vi "pickRobotsVSS.vi"(8 "error in (no error)":errorcluster, 11 "Game in":refnum<class "Game.lvclass">) -> (0 "error out":errorcluster, 3 "Game out":refnum<class "Game.lvclass">)   [LabVIEW 2020, in "Game.lvclass"]
uses:
  Game.lvclass
  Game.lvclass/Game.ctl
  Referee_class/Referee.lvclass/Referee.ctl
  Team_class/Team.lvclass/Team.ctl
  Robot_class/roles.ctl
  Robot_class/Robot.lvclass/Robot.ctl
  Role_class/Role.lvclass/Role.ctl
  HaltPlay_class/HaltPlay.lvclass/HaltPlay.ctl
  TimeoutPlay_class/TimeoutPlay.lvclass/TimeoutPlay.ctl
  Robot_class/Write role.vi
  Role_class/Write RobotRef.vi
  HaltPlay_class/Read Roles.vi
  HaltPlay_class/Write Roles.vi
  TimeoutPlay_class/Read Roles.vi
  TimeoutPlay_class/Write Roles.vi
  Read KeeperTeam.vi
  Read AllyRef.vi
  Read Referee.vi
  Read TestMode IDs.vi
  Referee_class/Read our_goalie_id.vi
  Team_class/Read RobotRef.vi
  Team_class/Write RobotRef.vi
  Write KeeperTeam.vi
  Ally_class/Ally.lvclass
  C:/Users/lucio/Desktop/Horie/ROBOIME/VSS_AI/Team_class/Team.lvclass
  KeeperRoleVSS_class/KeeperRoleVSS.lvclass
  C:/Users/lucio/Desktop/Horie/ROBOIME/VSS_AI/Role_class/Role.lvclass
  NormalAttackerRoleVSS_class/NormalAttackerRoleVSS.lvclass
  DefenderAreaRoleVSS_class/DefenderAreaRoleVSS.lvclass
  HaltRole_class/HaltRole.lvclass
  GoalKickKeeperRoleVSS_class/GoalKickKeeperRoleVSS.lvclass
  GoAndKickRoleVSS_class/GoAndKickRoleVSS.lvclass
  BallChallengerAttackerRoleVSS_class/BallChallengerAttackerRoleVSS.lvclass
  TimeoutRole_class/TimeoutRole.lvclass
  Referee_class/Referee.lvclass
  Playbook_class/Playbook.lvclass
  Robot_class/Robot.lvclass
  PreparePenaltyAllyPlayVSS_class/PreparePenaltyAllyPlayVSS.lvclass
  HaltPlay_class/HaltPlay.lvclass
  DeadBallPlayVSS_class/DeadBallPlayVSS.lvclass
  NormalGamePlayVSS_class/NormalGamePlayVSS.lvclass
  BallChallengePlayVSS_class/BallChallengePlayVSS.lvclass
  PenaltyEnemyPlayVSS_class/PenaltyEnemyPlayVSS.lvclass
  TimeoutPlay_class/TimeoutPlay.lvclass
  KickPenaltyAllyPlayVSS_class/KickPenaltyAllyPlayVSS.lvclass
  PreparePenaltyEnemyPlayVSS_class/PreparePenaltyEnemyPlayVSS.lvclass
  PrepareKickoffAllyPlayVSS_class/PrepareKickoffAllyPlayVSS.lvclass
  PrepareKickoffEnemyPlayVSS_class/PrepareKickoffEnemyPlayVSS.lvclass
  PrepareGoalKickAllyPlayVSS_class/PrepareGoalKickAllyPlayVSS.lvclass
  PrepareGoalKickEnemyPlayVSS_class/PrepareGoalKickEnemyPlayVSS.lvclass
  PrepareFreeBallPlayVSS_class/PrepareFreeBallPlayVSS.lvclass
  FreeBallPlayVSS_class/FreeBallPlayVSS.lvclass
  GoalKickAllyPlayVSS_class/GoalKickAllyPlayVSS.lvclass
  GoalKickEnemyPlayVSS_class/GoalKickEnemyPlayVSS.lvclass
  KickoffAllyPlayVSS_class/KickoffAllyPlayVSS.lvclass
  KickoffEnemyPlayVSS_class/KickoffEnemyPlayVSS.lvclass
  StopPlayVSS_class/StopPlayVSS.lvclass
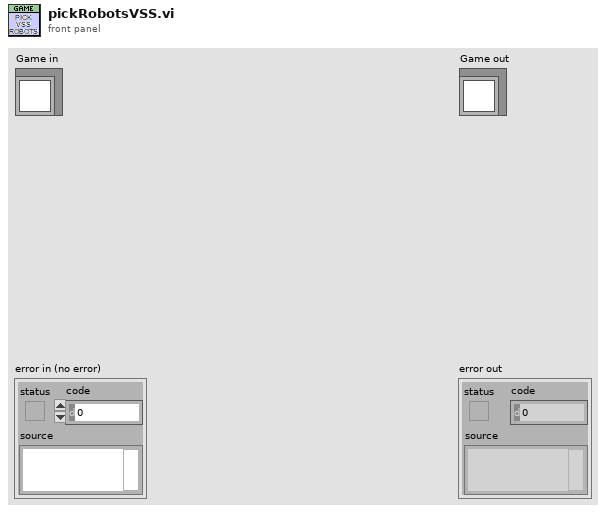
[diagram p1: front panel]
types:
  T1 = typedef "roles.ctl" = enum16{"BallChallengerAttackerVSS", "NormalAttackerVSS", "AttackerAimGoalVSS", "DefenderAreaVSS", "KeeperVSS", "Tabler", "TableFinalizer", "PrepareRollToPassRoller", "PrepareRollToPassReceiver", "SimplePassRoll", "SimplePassRollReceiver", "PenaltyDefense", "PreparePassReceiver 2", "PreparePassReceiver 1", "PassObserver", "Timeout", "Goto", "ZigZag", "None", "BallOutOfField", "DefenderArea", "Duelist", "AttackerStop", "FollowAttacker", "KeeperRole", "KickPenalty", "AttackerAimGoal", "AttackerBlock", "Marker", "Halt", "Shoot", "PassKicker", "PassReceiver", "TestRole", "PenaltyAttacker"}
  T2 = enum16{"FreeBall", "PrepareFreeBall", "GoalKickEnemy", "GoalKickAlly", "KickoffAlly", "KickoffEnemy", "PrepareGoalKickEnemy", "PrepareGoalKickAlly", "Stop", "PrepareKickoffEnemy", "PrepareKickoffAlly", "PreparePenaltyEnemy", "Timeout", "DeadBall", "NormalGame", "KickPenaltyAlly", "PenaltyEnemy", "BallChallenge", "PreparePenaltyAlly", "Halt"}
  T3 = cluster{"PreparePenaltyAllyPlayVSS":refnum<class "PreparePenaltyAllyPlayVSS.lvclass">, "HaltPlay":refnum<class "HaltPlay.lvclass">, "DeadBallPlayVSS":refnum<class "DeadBallPlayVSS.lvclass">, "NormalGamePlayVSS":refnum<class "NormalGamePlayVSS.lvclass">, "BallChallengePlayVSS":refnum<class "BallChallengePlayVSS.lvclass">, "PenaltyEnemyPlayVSS":refnum<class "PenaltyEnemyPlayVSS.lvclass">, "TimeoutPlay":refnum<class "TimeoutPlay.lvclass">, "KickPenaltyAllyPlayVSS":refnum<class "KickPenaltyAllyPlayVSS.lvclass">, "PreparePenaltyEnemyPlayVSS":refnum<class "PreparePenaltyEnemyPlayVSS.lvclass">, "PrepareKickoffAllyPlayVSS":refnum<class "PrepareKickoffAllyPlayVSS.lvclass">, "PrepareKickoffEnemyPlayVSS":refnum<class "PrepareKickoffEnemyPlayVSS.lvclass">, "PrepareGoalKickAllyPlayVSS":refnum<class "PrepareGoalKickAllyPlayVSS.lvclass">, "PrepareGoalKickEnemyPlayVSS":refnum<class "PrepareGoalKickEnemyPlayVSS.lvclass">, "PrepareFreeBallPlayVSS":refnum<class "PrepareFreeBallPlayVSS.lvclass">, "FreeBallPlayVSS":refnum<class "FreeBallPlayVSS.lvclass">, "GoalKickAllyPlayVSS":refnum<class "GoalKickAllyPlayVSS.lvclass">, "GoalKickEnemyPlayVSS":refnum<class "GoalKickEnemyPlayVSS.lvclass">, "KickoffAllyPlayVSS":refnum<class "KickoffAllyPlayVSS.lvclass">, "KickoffEnemyPlayVSS":refnum<class "KickoffEnemyPlayVSS.lvclass">, "StopPlayVSS":refnum<class "StopPlayVSS.lvclass">}
  T4 = cluster{"NormalAttackerRoleVSS":refnum<class "NormalAttackerRoleVSS.lvclass">, "KeeperRoleVSS":refnum<class "KeeperRoleVSS.lvclass">, "DefenderAreaRoleVSS":refnum<class "DefenderAreaRoleVSS.lvclass">}
  T5 = cluster{"HaltRole K":refnum<class "HaltRole.lvclass">, "HaltRole D":refnum<class "HaltRole.lvclass">, "HaltRole A":refnum<class "HaltRole.lvclass">}
  T6 = cluster{"KeeperRoleVSS":refnum<class "KeeperRoleVSS.lvclass">, "DefenderAreaRoleVSS":refnum<class "DefenderAreaRoleVSS.lvclass">, "HaltRole":refnum<class "HaltRole.lvclass">}
  T7 = cluster{"HaltRole A":refnum<class "HaltRole.lvclass">, "HaltRole D":refnum<class "HaltRole.lvclass">, "GoalKickKeeperRoleVSS":refnum<class "GoalKickKeeperRoleVSS.lvclass">}
  T8 = cluster{"KeeperRoleVSS":refnum<class "KeeperRoleVSS.lvclass">, "HaltRole":refnum<class "HaltRole.lvclass">, "GoAndKickRoleVSS":refnum<class "GoAndKickRoleVSS.lvclass">}
  T9 = cluster{"KeeperRoleVSS":refnum<class "KeeperRoleVSS.lvclass">, "HaltRole A":refnum<class "HaltRole.lvclass">, "HaltRole D":refnum<class "HaltRole.lvclass">}
  T10 = cluster{"HaltRole 1":refnum<class "HaltRole.lvclass">, "HaltRole 2":refnum<class "HaltRole.lvclass">, "HaltRole 3":refnum<class "HaltRole.lvclass">, "HaltRole 4":refnum<class "HaltRole.lvclass">, "HaltRole 5":refnum<class "HaltRole.lvclass">, "HaltRole 6":refnum<class "HaltRole.lvclass">}
  T11 = cluster{"NormalAttackerRoleVSS":refnum<class "NormalAttackerRoleVSS.lvclass">, "HaltRole K":refnum<class "HaltRole.lvclass">, "HaltRole D":refnum<class "HaltRole.lvclass">}
  T12 = cluster{"HaltRole 1":refnum<class "HaltRole.lvclass">, "HaltRole 2":refnum<class "HaltRole.lvclass">, "BallChallengerAttackerRoleVSS":refnum<class "BallChallengerAttackerRoleVSS.lvclass">}
  T13 = cluster{"TimeoutRole 1":refnum<class "TimeoutRole.lvclass">, "TimeoutRole 2":refnum<class "TimeoutRole.lvclass">, "TimeoutRole 3":refnum<class "TimeoutRole.lvclass">, "TimeoutRole 4":refnum<class "TimeoutRole.lvclass">, "TimeoutRole 5":refnum<class "TimeoutRole.lvclass">, "TimeoutRole 6":refnum<class "TimeoutRole.lvclass">}
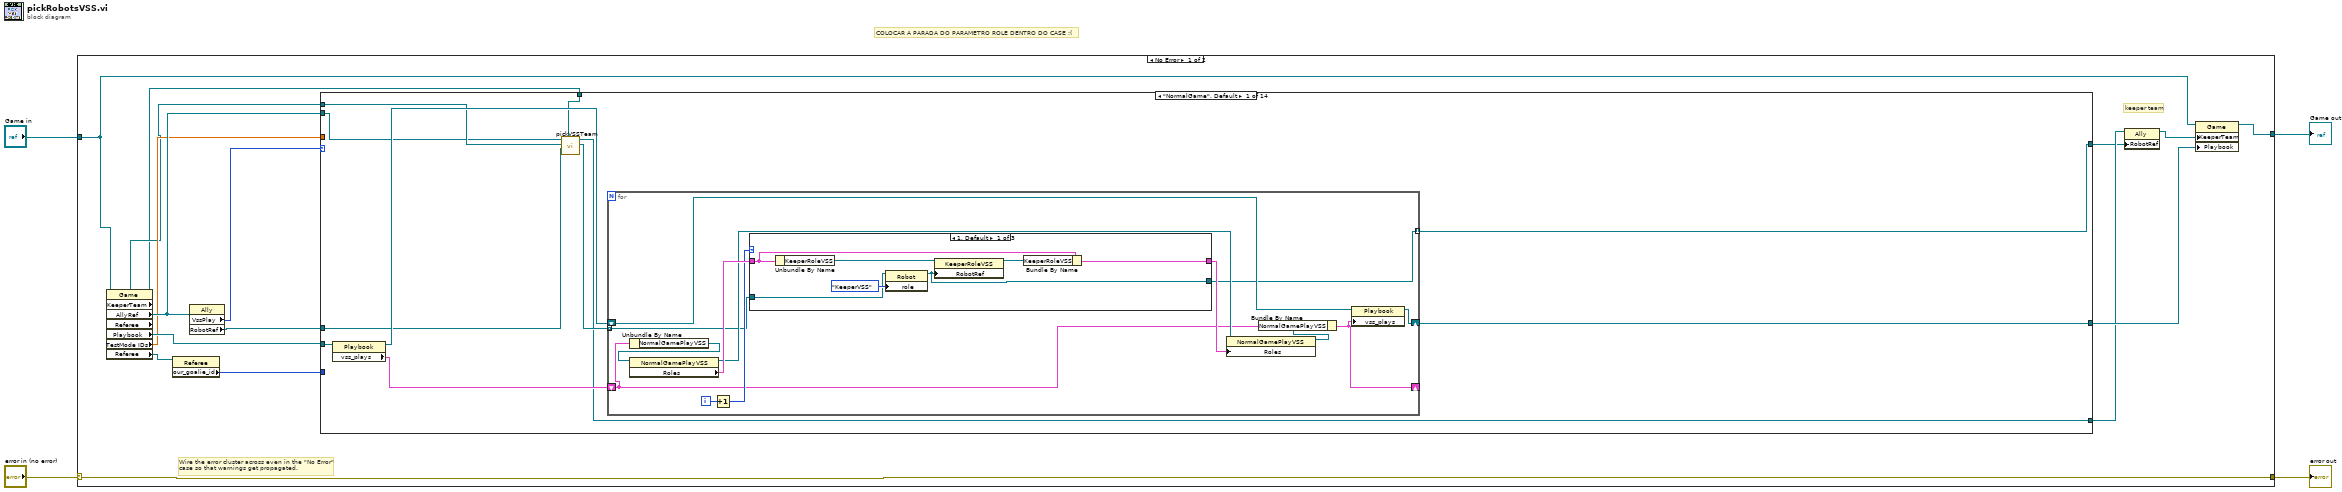
[diagram p0: block diagram]
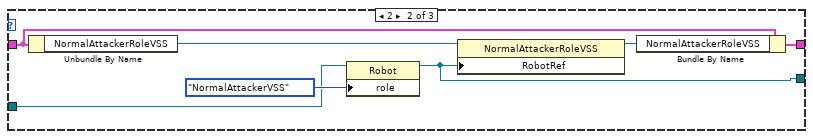
[diagram p2: hidden frame]
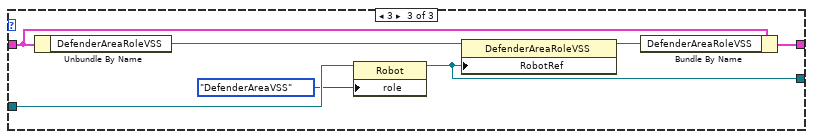
[diagram p3: hidden frame]
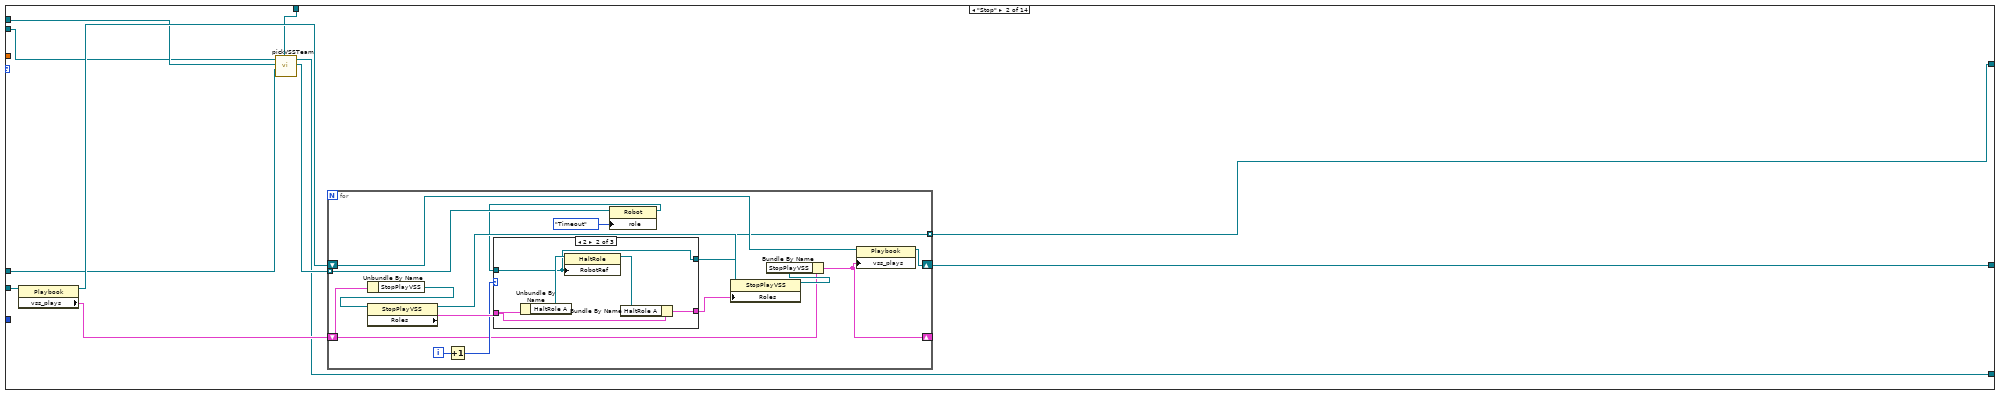
[diagram p4: hidden frame]
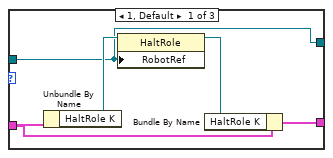
[diagram p5: hidden frame]
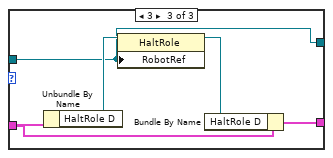
[diagram p6: hidden frame]
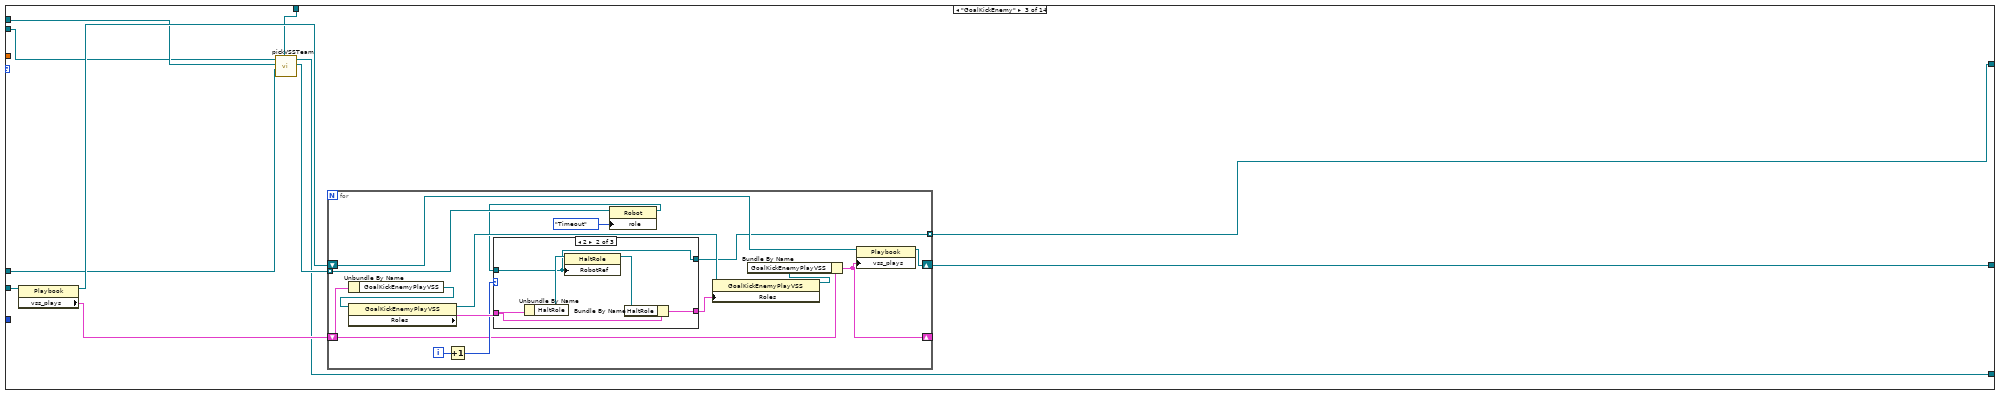
[diagram p7: hidden frame]
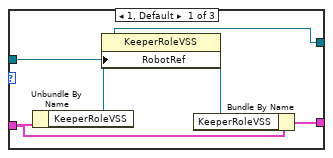
[diagram p8: hidden frame]
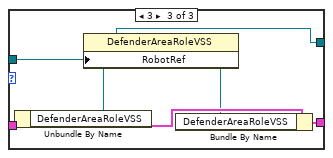
[diagram p9: hidden frame]
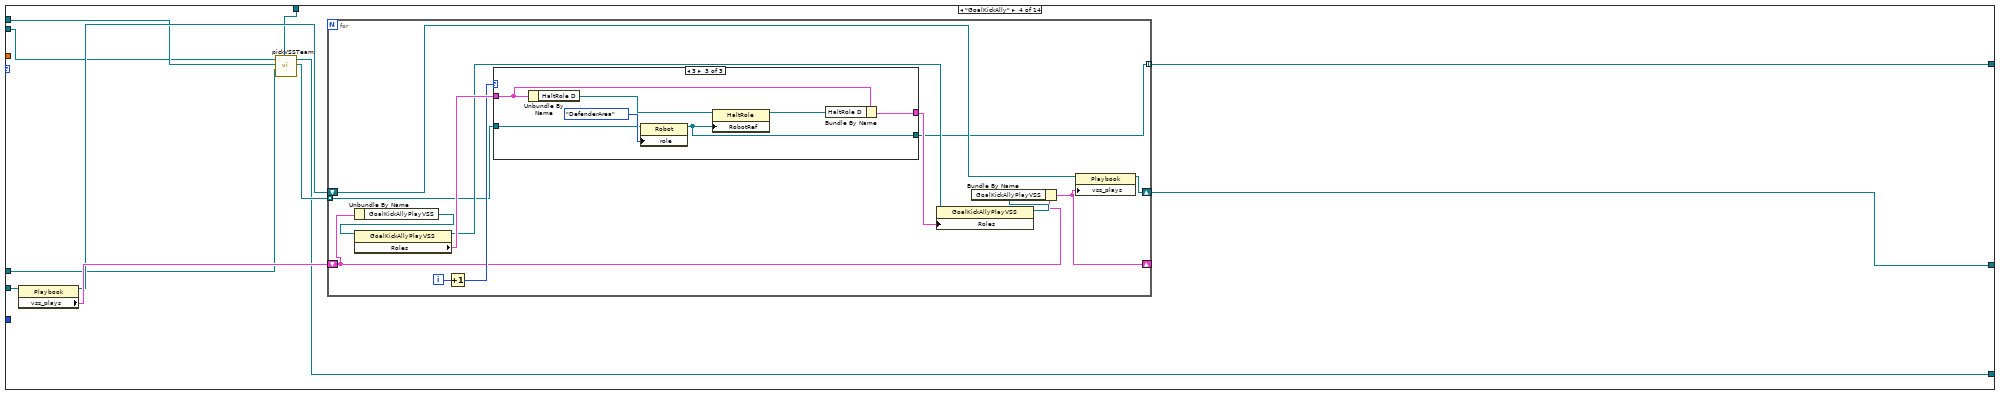
[diagram p10: hidden frame]
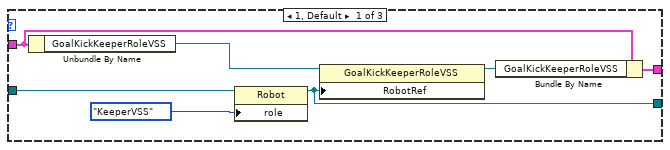
[diagram p11: hidden frame]
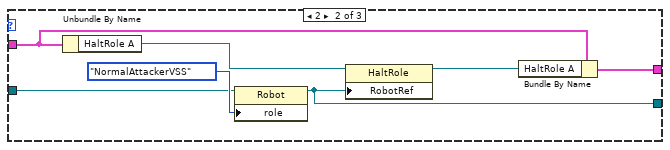
[diagram p12: hidden frame]
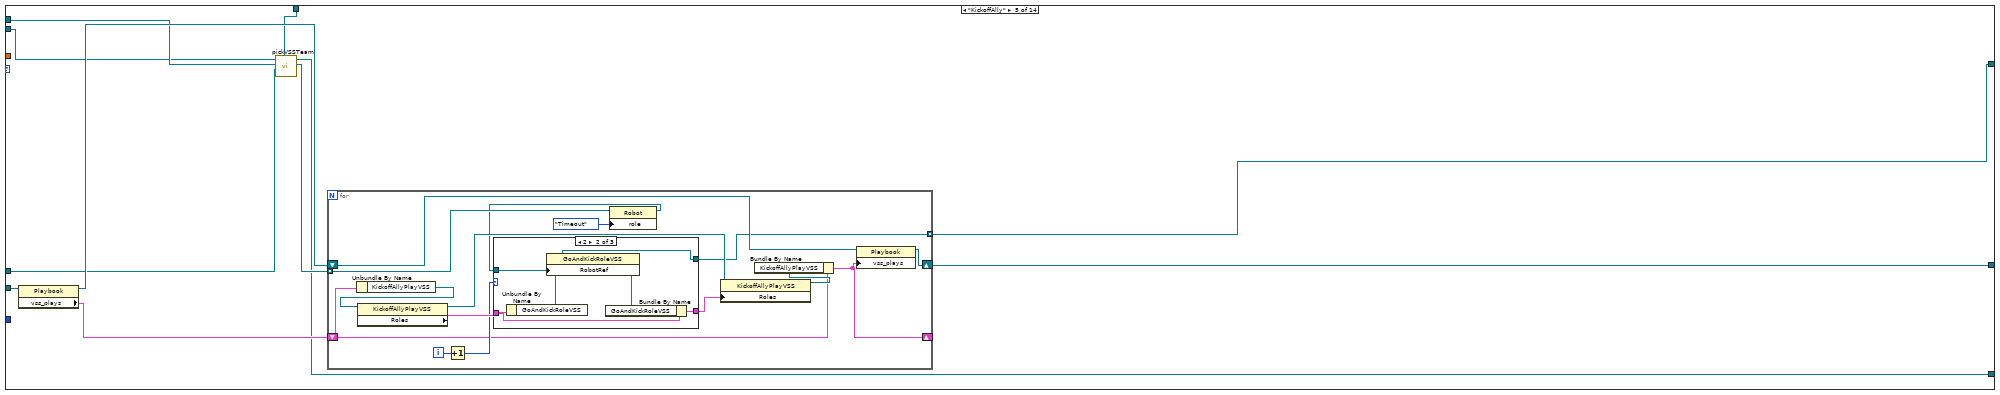
[diagram p13: hidden frame]
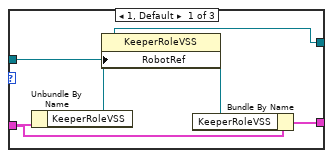
[diagram p14: hidden frame]
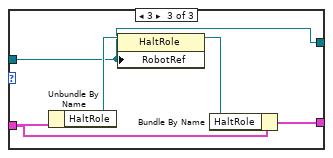
[diagram p15: hidden frame]
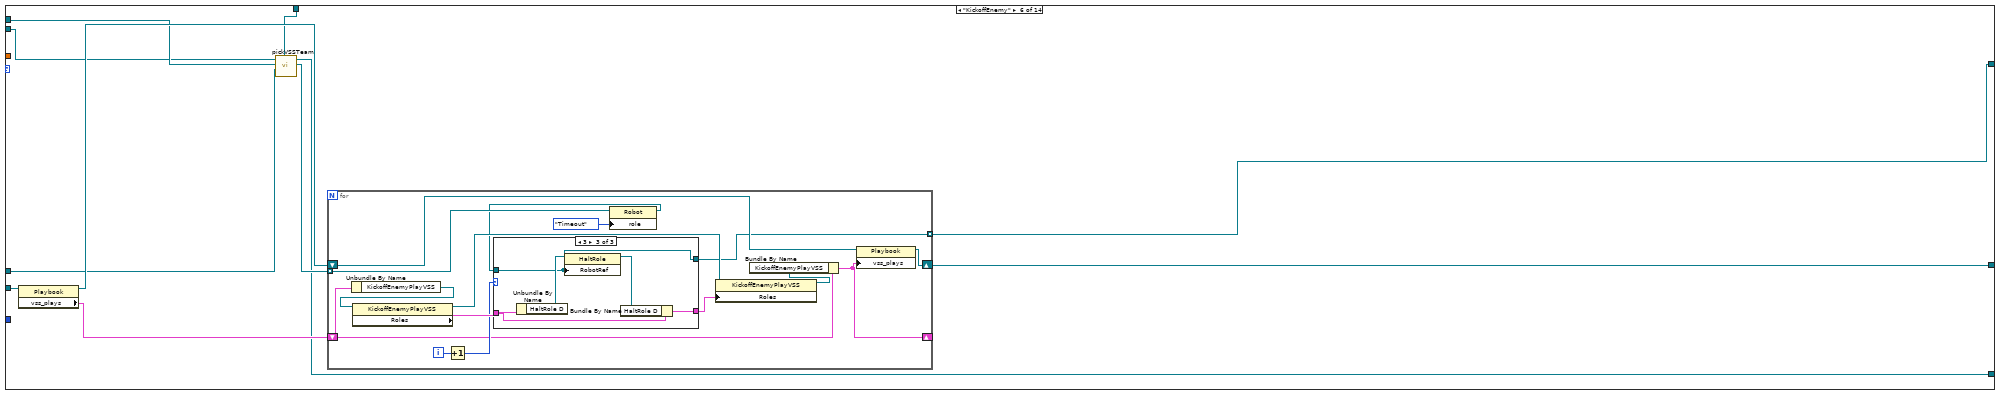
[diagram p16: hidden frame]
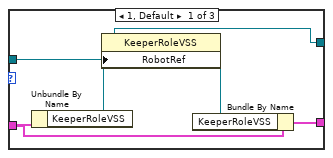
[diagram p17: hidden frame]
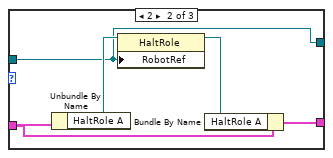
[diagram p18: hidden frame]
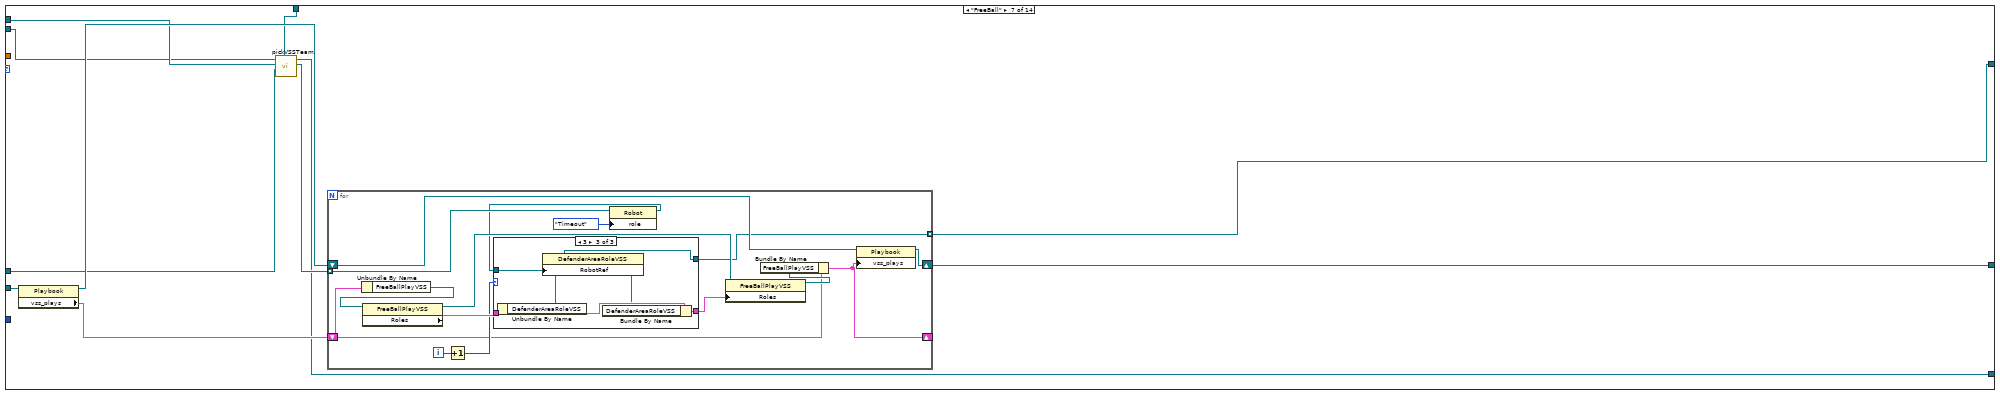
[diagram p19: hidden frame]
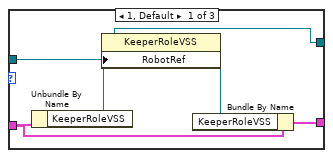
[diagram p20: hidden frame]
diagram:
  # "COLOCAR A PARADA DO PARAMETRO ROLE DENTRO DO CASE :("
  n1 = case shown="No Error" "error in (no error)" {
    selector: "error in (no error)" -> [w15 w604]
    tunnel: [w15 w604] -> w3
    tunnel: [w16 w603] -> w1
    tunnel: "Game in" -> [w18 w603]
    frame No Error {
      # "keeper team"
      # "Wire the error cluster across even in the \"No Error\"\ncase so that warnings get propagated."
      n2 = property class="Game" props=["KeeperTeam", "AllyRef", "Referee", "Playbook", "TestMode IDs", "Referee"](reference=w18) -> (reference out=w5:refnum<class "Game.lvclass">, "KeeperTeam"=w6:refnum<class "Ally.lvclass">, "AllyRef"=w12:refnum<class "Ally.lvclass">, "Playbook"=w20:refnum<class "Playbook.lvclass">, "TestMode IDs"=w9:dbl[], "Referee"=w8:refnum<class "Referee.lvclass">)  [unwired: 1 in, 2 out]
      n3 = property class="Referee"(reference=w8) -> ("our_goalie_id"=w7:i32)  [unwired: 1 in, 2 out]
      n4 = property class="Ally"(reference=w12) -> ("VssPlay"=w10:T2, "RobotRef"=w19:refnum<class "Robot.lvclass">[])  [unwired: 1 in, 2 out]
      n5 = case shown="\"NormalGame\", Default" w10 {
        tunnel: w20 -> [w31 w76 w117 w158 w203 w244 w285 w326 w367 w408 w449 w490 w531 w572]
        tunnel: w19 -> [w24 w69 w110 w151 w196 w237 w278 w319 w360 w401 w442 w483 w524 w565]
        tunnel: [w29 w74 w115 w156 w201 w242 w283 w324 w365 w406 w447 w488 w529 w570] -> w17
        tunnel: [w28 w73 w114 w155 w200 w241 w282 w323 w364 w405 w446 w487 w528 w569] -> w11
        tunnel: [w21 w66 w107 w148 w193 w234 w275 w316 w357 w398 w439 w480 w521 w562] -> w13
        tunnel: w12 -> [w25 w70 w111 w152 w197 w238 w279 w320 w361 w402 w443 w484 w525 w566]
        tunnel: w9 -> [_ _ _ _ _ _ _ _ _ _ _ _ _ _]
        tunnel: w7 -> [_ _ _ _ _ _ _ _ _ _ _ _ _ _]
        tunnel: w6 -> [w26 w71 w112 w153 w198 w239 w280 w321 w362 w403 w444 w485 w526 w567]
        tunnel: w5 -> [w23 w68 w109 w150 w195 w236 w277 w318 w359 w400 w441 w482 w523 w564]
        frame "NormalGame", Default {
          n6 = property class="Playbook"(reference=w31) -> (reference out=w27:refnum<class "Playbook.lvclass">, "vss_plays"=w30:T3)  [unwired: 1 in, 1 out]
          n7 = call "pickVSSTeam.vi"("Ally in"=w25, "OldVSSTeam"=w26, "RobotRef"=w24, "Game"=w23) -> ("Ally out"=w21:refnum<class "Ally.lvclass">, "RobotRef Out"=w22:refnum<class "Robot.lvclass">[])  [unwired: 4 in, 1 out]
          n8 = for {
            tunnel: [w34] -> w28 mode=indexing
            tunnel: w22 -> [w32] mode=indexing
            shift-right: [w39] -> w29
            shift-left: w27 -> [w40]
            shift-right: [w33] -> _
            shift-left: w30 -> [w36]
            i -> [w38]
            n9 = Unbundle By Name(w36) -> ("NormalGamePlayVSS"=w35:refnum<class "NormalGamePlayVSS.lvclass">)
            n10 = property class="NormalGamePlayVSS"(reference=w35) -> (reference out=w42:refnum<class "NormalGamePlayVSS.lvclass">, "Roles"=w44:T4)  [unwired: 1 in, 1 out]
            n11 = Increment(x=w38) -> (x+1=w37:i32)
            n12 = case shown="1, Default" w37 {
              tunnel: w44 -> [w50 w57 w64]
              tunnel: [w49 w56 w63] -> w43
              tunnel: [w45 w52 w61] -> w34
              tunnel: w32 -> [w46 w53 w60]
              frame 1, Default {
                n13 = Unbundle By Name(w50) -> ("KeeperRoleVSS"=w51:refnum<class "KeeperRoleVSS.lvclass">)
                n14 = property class="Robot"(reference=w46, "role"=roles."KeeperVSS") -> (reference out=w45:refnum<class "Robot.lvclass">)  [unwired: 1 in, 1 out]
                n15 = property class="KeeperRoleVSS"(reference=w51, "RobotRef"=w45) -> (reference out=w48:refnum<class "KeeperRoleVSS.lvclass">)  [unwired: 1 in, 1 out]
                n16 = Bundle By Name(cluster=w50, "KeeperRoleVSS"=w48) -> (w49:T4)
              }
              frame 2 {
                n17 = Unbundle By Name(w57) -> ("NormalAttackerRoleVSS"=w58:refnum<class "NormalAttackerRoleVSS.lvclass">)
                n18 = property class="Robot"(reference=w53, "role"=roles."NormalAttackerVSS") -> (reference out=w52:refnum<class "Robot.lvclass">)  [unwired: 1 in, 1 out]
                n19 = property class="NormalAttackerRoleVSS"(reference=w58, "RobotRef"=w52) -> (reference out=w55:refnum<class "NormalAttackerRoleVSS.lvclass">)  [unwired: 1 in, 1 out]
                n20 = Bundle By Name(cluster=w57, "NormalAttackerRoleVSS"=w55) -> (w56:T4)
              }
              frame 3 {
                n21 = Unbundle By Name(w64) -> ("DefenderAreaRoleVSS"=w65:refnum<class "DefenderAreaRoleVSS.lvclass">)
                n22 = property class="Robot"(reference=w60, "role"=roles."DefenderAreaVSS") -> (reference out=w61:refnum<class "Robot.lvclass">)  [unwired: 1 in, 1 out]
                n23 = property class="DefenderAreaRoleVSS"(reference=w65, "RobotRef"=w61) -> (reference out=w62:refnum<class "DefenderAreaRoleVSS.lvclass">)  [unwired: 1 in, 1 out]
                n24 = Bundle By Name(cluster=w64, "DefenderAreaRoleVSS"=w62) -> (w63:T4)
              }
            }
            n25 = property class="NormalGamePlayVSS"(reference=w42, "Roles"=w43) -> (reference out=w41:refnum<class "NormalGamePlayVSS.lvclass">)  [unwired: 1 in, 1 out]
            n26 = Bundle By Name(cluster=w36, "NormalGamePlayVSS"=w41) -> (w33:T3)
            n27 = property class="Playbook"(reference=w40, "vss_plays"=w33) -> (reference out=w39:refnum<class "Playbook.lvclass">)  [unwired: 1 in, 1 out]
          }
        }
        frame "Stop" {
          n28 = property class="Playbook"(reference=w76) -> (reference out=w72:refnum<class "Playbook.lvclass">, "vss_plays"=w75:T3)  [unwired: 1 in, 1 out]
          n29 = call "pickVSSTeam.vi"("Ally in"=w70, "OldVSSTeam"=w71, "RobotRef"=w69, "Game"=w68) -> ("Ally out"=w66:refnum<class "Ally.lvclass">, "RobotRef Out"=w67:refnum<class "Robot.lvclass">[])  [unwired: 4 in, 1 out]
          n30 = for {
            tunnel: [w79] -> w73 mode=indexing
            tunnel: w67 -> [w84] mode=indexing
            shift-right: [w86] -> w74
            shift-left: w72 -> [w87]
            shift-right: [w77] -> _
            shift-left: w75 -> [w81]
            i -> [w83]
            n31 = Unbundle By Name(w81) -> ("StopPlayVSS"=w80:refnum<class "StopPlayVSS.lvclass">)
            n32 = property class="StopPlayVSS"(reference=w80) -> (reference out=w89:refnum<class "StopPlayVSS.lvclass">, "Roles"=w91:T5)  [unwired: 1 in, 1 out]
            n33 = Increment(x=w83) -> (x+1=w82:i32)
            n34 = property class="Robot"(reference=w84, "role"=roles."Timeout") -> (reference out=w78:refnum<class "Robot.lvclass">)  [unwired: 1 in, 1 out]
            n35 = case shown="2" w82 {
              tunnel: w91 -> [w95 w100 w105]
              tunnel: [w94 w99 w104] -> w90
              tunnel: w78 -> [w92 w97 w102]
              tunnel: [w92 w97 w102] -> w79
              frame 1, Default {
                n36 = Unbundle By Name(w95) -> ("HaltRole K"=w96:refnum<class "HaltRole.lvclass">)
                n37 = property class="HaltRole"(reference=w96, "RobotRef"=w92) -> (reference out=w93:refnum<class "HaltRole.lvclass">)  [unwired: 1 in, 1 out]
                n38 = Bundle By Name(cluster=w95, "HaltRole K"=w93) -> (w94:T5)
              }
              frame 2 {
                n39 = Unbundle By Name(w100) -> ("HaltRole A"=w101:refnum<class "HaltRole.lvclass">)
                n40 = property class="HaltRole"(reference=w101, "RobotRef"=w97) -> (reference out=w98:refnum<class "HaltRole.lvclass">)  [unwired: 1 in, 1 out]
                n41 = Bundle By Name(cluster=w100, "HaltRole A"=w98) -> (w99:T5)
              }
              frame 3 {
                n42 = Unbundle By Name(w105) -> ("HaltRole D"=w106:refnum<class "HaltRole.lvclass">)
                n43 = property class="HaltRole"(reference=w106, "RobotRef"=w102) -> (reference out=w103:refnum<class "HaltRole.lvclass">)  [unwired: 1 in, 1 out]
                n44 = Bundle By Name(cluster=w105, "HaltRole D"=w103) -> (w104:T5)
              }
            }
            n45 = property class="StopPlayVSS"(reference=w89, "Roles"=w90) -> (reference out=w88:refnum<class "StopPlayVSS.lvclass">)  [unwired: 1 in, 1 out]
            n46 = Bundle By Name(cluster=w81, "StopPlayVSS"=w88) -> (w77:T3)
            n47 = property class="Playbook"(reference=w87, "vss_plays"=w77) -> (reference out=w86:refnum<class "Playbook.lvclass">)  [unwired: 1 in, 1 out]
          }
        }
        frame "GoalKickEnemy" {
          n48 = property class="Playbook"(reference=w117) -> (reference out=w113:refnum<class "Playbook.lvclass">, "vss_plays"=w116:T3)  [unwired: 1 in, 1 out]
          n49 = call "pickVSSTeam.vi"("Ally in"=w111, "OldVSSTeam"=w112, "RobotRef"=w110, "Game"=w109) -> ("Ally out"=w107:refnum<class "Ally.lvclass">, "RobotRef Out"=w108:refnum<class "Robot.lvclass">[])  [unwired: 4 in, 1 out]
          n50 = for {
            tunnel: [w120] -> w114 mode=indexing
            tunnel: w108 -> [w125] mode=indexing
            shift-right: [w127] -> w115
            shift-left: w113 -> [w128]
            shift-right: [w118] -> _
            shift-left: w116 -> [w122]
            i -> [w124]
            n51 = Unbundle By Name(w122) -> ("GoalKickEnemyPlayVSS"=w121:refnum<class "GoalKickEnemyPlayVSS.lvclass">)
            n52 = property class="GoalKickEnemyPlayVSS"(reference=w121) -> (reference out=w130:refnum<class "GoalKickEnemyPlayVSS.lvclass">, "Roles"=w132:T6)  [unwired: 1 in, 1 out]
            n53 = Increment(x=w124) -> (x+1=w123:i32)
            n54 = property class="Robot"(reference=w125, "role"=roles."Timeout") -> (reference out=w119:refnum<class "Robot.lvclass">)  [unwired: 1 in, 1 out]
            n55 = case shown="2" w123 {
              tunnel: w132 -> [w136 w141 w146]
              tunnel: [w135 w140 w145] -> w131
              tunnel: w119 -> [w133 w138 w143]
              tunnel: [w133 w138 w143] -> w120
              frame 1, Default {
                n56 = Unbundle By Name(w136) -> ("KeeperRoleVSS"=w137:refnum<class "KeeperRoleVSS.lvclass">)
                n57 = property class="KeeperRoleVSS"(reference=w137, "RobotRef"=w133) -> (reference out=w134:refnum<class "KeeperRoleVSS.lvclass">)  [unwired: 1 in, 1 out]
                n58 = Bundle By Name(cluster=w136, "KeeperRoleVSS"=w134) -> (w135:T6)
              }
              frame 2 {
                n59 = Unbundle By Name(w141) -> ("HaltRole"=w142:refnum<class "HaltRole.lvclass">)
                n60 = property class="HaltRole"(reference=w142, "RobotRef"=w138) -> (reference out=w139:refnum<class "HaltRole.lvclass">)  [unwired: 1 in, 1 out]
                n61 = Bundle By Name(cluster=w141, "HaltRole"=w139) -> (w140:T6)
              }
              frame 3 {
                n62 = Unbundle By Name(w146) -> ("DefenderAreaRoleVSS"=w147:refnum<class "DefenderAreaRoleVSS.lvclass">)
                n63 = property class="DefenderAreaRoleVSS"(reference=w147, "RobotRef"=w143) -> (reference out=w144:refnum<class "DefenderAreaRoleVSS.lvclass">)  [unwired: 1 in, 1 out]
                n64 = Bundle By Name(cluster=w146, "DefenderAreaRoleVSS"=w144) -> (w145:T6)
              }
            }
            n65 = property class="GoalKickEnemyPlayVSS"(reference=w130, "Roles"=w131) -> (reference out=w129:refnum<class "GoalKickEnemyPlayVSS.lvclass">)  [unwired: 1 in, 1 out]
            n66 = Bundle By Name(cluster=w122, "GoalKickEnemyPlayVSS"=w129) -> (w118:T3)
            n67 = property class="Playbook"(reference=w128, "vss_plays"=w118) -> (reference out=w127:refnum<class "Playbook.lvclass">)  [unwired: 1 in, 1 out]
          }
        }
        frame "GoalKickAlly" {
          n68 = property class="Playbook"(reference=w158) -> (reference out=w154:refnum<class "Playbook.lvclass">, "vss_plays"=w157:T3)  [unwired: 1 in, 1 out]
          n69 = call "pickVSSTeam.vi"("Ally in"=w152, "OldVSSTeam"=w153, "RobotRef"=w151, "Game"=w150) -> ("Ally out"=w148:refnum<class "Ally.lvclass">, "RobotRef Out"=w149:refnum<class "Robot.lvclass">[])  [unwired: 4 in, 1 out]
          n70 = for {
            tunnel: [w161] -> w155 mode=indexing
            tunnel: w149 -> [w159] mode=indexing
            shift-right: [w166] -> w156
            shift-left: w154 -> [w167]
            shift-right: [w160] -> _
            shift-left: w157 -> [w163]
            i -> [w165]
            n71 = Unbundle By Name(w163) -> ("GoalKickAllyPlayVSS"=w162:refnum<class "GoalKickAllyPlayVSS.lvclass">)
            n72 = property class="GoalKickAllyPlayVSS"(reference=w162) -> (reference out=w169:refnum<class "GoalKickAllyPlayVSS.lvclass">, "Roles"=w171:T7)  [unwired: 1 in, 1 out]
            n73 = Increment(x=w165) -> (x+1=w164:i32)
            n74 = case shown="3" w164 {
              tunnel: w171 -> [w177 w184 w191]
              tunnel: [w176 w183 w190] -> w170
              tunnel: [w174 w179 w186] -> w161
              tunnel: w159 -> [w173 w180 w187]
              frame 1, Default {
                n75 = Unbundle By Name(w177) -> ("GoalKickKeeperRoleVSS"=w178:refnum<class "GoalKickKeeperRoleVSS.lvclass">)
                n76 = property class="Robot"(reference=w173, "role"=roles."KeeperVSS") -> (reference out=w174:refnum<class "Robot.lvclass">)  [unwired: 1 in, 1 out]
                n77 = property class="GoalKickKeeperRoleVSS"(reference=w178, "RobotRef"=w174) -> (reference out=w175:refnum<class "GoalKickKeeperRoleVSS.lvclass">)  [unwired: 1 in, 1 out]
                n78 = Bundle By Name(cluster=w177, "GoalKickKeeperRoleVSS"=w175) -> (w176:T7)
              }
              frame 2 {
                n79 = Unbundle By Name(w184) -> ("HaltRole A"=w185:refnum<class "HaltRole.lvclass">)
                n80 = property class="Robot"(reference=w180, "role"=roles."NormalAttackerVSS") -> (reference out=w179:refnum<class "Robot.lvclass">)  [unwired: 1 in, 1 out]
                n81 = property class="HaltRole"(reference=w185, "RobotRef"=w179) -> (reference out=w182:refnum<class "HaltRole.lvclass">)  [unwired: 1 in, 1 out]
                n82 = Bundle By Name(cluster=w184, "HaltRole A"=w182) -> (w183:T7)
              }
              frame 3 {
                n83 = Unbundle By Name(w191) -> ("HaltRole D"=w192:refnum<class "HaltRole.lvclass">)
                n84 = property class="Robot"(reference=w187, "role"=roles."DefenderArea") -> (reference out=w186:refnum<class "Robot.lvclass">)  [unwired: 1 in, 1 out]
                n85 = property class="HaltRole"(reference=w192, "RobotRef"=w186) -> (reference out=w189:refnum<class "HaltRole.lvclass">)  [unwired: 1 in, 1 out]
                n86 = Bundle By Name(cluster=w191, "HaltRole D"=w189) -> (w190:T7)
              }
            }
            n87 = property class="GoalKickAllyPlayVSS"(reference=w169, "Roles"=w170) -> (reference out=w168:refnum<class "GoalKickAllyPlayVSS.lvclass">)  [unwired: 1 in, 1 out]
            n88 = Bundle By Name(cluster=w163, "GoalKickAllyPlayVSS"=w168) -> (w160:T3)
            n89 = property class="Playbook"(reference=w167, "vss_plays"=w160) -> (reference out=w166:refnum<class "Playbook.lvclass">)  [unwired: 1 in, 1 out]
          }
        }
        frame "KickoffAlly" {
          n90 = property class="Playbook"(reference=w203) -> (reference out=w199:refnum<class "Playbook.lvclass">, "vss_plays"=w202:T3)  [unwired: 1 in, 1 out]
          n91 = call "pickVSSTeam.vi"("Ally in"=w197, "OldVSSTeam"=w198, "RobotRef"=w196, "Game"=w195) -> ("Ally out"=w193:refnum<class "Ally.lvclass">, "RobotRef Out"=w194:refnum<class "Robot.lvclass">[])  [unwired: 4 in, 1 out]
          n92 = for {
            tunnel: [w206] -> w200 mode=indexing
            tunnel: w194 -> [w211] mode=indexing
            shift-right: [w213] -> w201
            shift-left: w199 -> [w214]
            shift-right: [w204] -> _
            shift-left: w202 -> [w208]
            i -> [w210]
            n93 = Unbundle By Name(w208) -> ("KickoffAllyPlayVSS"=w207:refnum<class "KickoffAllyPlayVSS.lvclass">)
            n94 = property class="KickoffAllyPlayVSS"(reference=w207) -> (reference out=w216:refnum<class "KickoffAllyPlayVSS.lvclass">, "Roles"=w218:T8)  [unwired: 1 in, 1 out]
            n95 = Increment(x=w210) -> (x+1=w209:i32)
            n96 = property class="Robot"(reference=w211, "role"=roles."Timeout") -> (reference out=w205:refnum<class "Robot.lvclass">)  [unwired: 1 in, 1 out]
            n97 = case shown="2" w209 {
              tunnel: w218 -> [w222 w227 w232]
              tunnel: [w221 w226 w231] -> w217
              tunnel: w205 -> [w219 w224 w229]
              tunnel: [w219 w224 w229] -> w206
              frame 1, Default {
                n98 = Unbundle By Name(w222) -> ("KeeperRoleVSS"=w223:refnum<class "KeeperRoleVSS.lvclass">)
                n99 = property class="KeeperRoleVSS"(reference=w223, "RobotRef"=w219) -> (reference out=w220:refnum<class "KeeperRoleVSS.lvclass">)  [unwired: 1 in, 1 out]
                n100 = Bundle By Name(cluster=w222, "KeeperRoleVSS"=w220) -> (w221:T8)
              }
              frame 2 {
                n101 = Unbundle By Name(w227) -> ("GoAndKickRoleVSS"=w228:refnum<class "GoAndKickRoleVSS.lvclass">)
                n102 = property class="GoAndKickRoleVSS"(reference=w228, "RobotRef"=w224) -> (reference out=w225:refnum<class "GoAndKickRoleVSS.lvclass">)  [unwired: 1 in, 1 out]
                n103 = Bundle By Name(cluster=w227, "GoAndKickRoleVSS"=w225) -> (w226:T8)
              }
              frame 3 {
                n104 = Unbundle By Name(w232) -> ("HaltRole"=w233:refnum<class "HaltRole.lvclass">)
                n105 = property class="HaltRole"(reference=w233, "RobotRef"=w229) -> (reference out=w230:refnum<class "HaltRole.lvclass">)  [unwired: 1 in, 1 out]
                n106 = Bundle By Name(cluster=w232, "HaltRole"=w230) -> (w231:T8)
              }
            }
            n107 = property class="KickoffAllyPlayVSS"(reference=w216, "Roles"=w217) -> (reference out=w215:refnum<class "KickoffAllyPlayVSS.lvclass">)  [unwired: 1 in, 1 out]
            n108 = Bundle By Name(cluster=w208, "KickoffAllyPlayVSS"=w215) -> (w204:T3)
            n109 = property class="Playbook"(reference=w214, "vss_plays"=w204) -> (reference out=w213:refnum<class "Playbook.lvclass">)  [unwired: 1 in, 1 out]
          }
        }
        frame "KickoffEnemy" {
          n110 = property class="Playbook"(reference=w244) -> (reference out=w240:refnum<class "Playbook.lvclass">, "vss_plays"=w243:T3)  [unwired: 1 in, 1 out]
          n111 = call "pickVSSTeam.vi"("Ally in"=w238, "OldVSSTeam"=w239, "RobotRef"=w237, "Game"=w236) -> ("Ally out"=w234:refnum<class "Ally.lvclass">, "RobotRef Out"=w235:refnum<class "Robot.lvclass">[])  [unwired: 4 in, 1 out]
          n112 = for {
            tunnel: [w247] -> w241 mode=indexing
            tunnel: w235 -> [w252] mode=indexing
            shift-right: [w254] -> w242
            shift-left: w240 -> [w255]
            shift-right: [w245] -> _
            shift-left: w243 -> [w249]
            i -> [w251]
            n113 = Unbundle By Name(w249) -> ("KickoffEnemyPlayVSS"=w248:refnum<class "KickoffEnemyPlayVSS.lvclass">)
            n114 = property class="KickoffEnemyPlayVSS"(reference=w248) -> (reference out=w257:refnum<class "KickoffEnemyPlayVSS.lvclass">, "Roles"=w259:T9)  [unwired: 1 in, 1 out]
            n115 = Increment(x=w251) -> (x+1=w250:i32)
            n116 = property class="Robot"(reference=w252, "role"=roles."Timeout") -> (reference out=w246:refnum<class "Robot.lvclass">)  [unwired: 1 in, 1 out]
            n117 = case shown="3" w250 {
              tunnel: w259 -> [w263 w268 w273]
              tunnel: [w262 w267 w272] -> w258
              tunnel: w246 -> [w260 w265 w270]
              tunnel: [w260 w265 w270] -> w247
              frame 1, Default {
                n118 = Unbundle By Name(w263) -> ("KeeperRoleVSS"=w264:refnum<class "KeeperRoleVSS.lvclass">)
                n119 = property class="KeeperRoleVSS"(reference=w264, "RobotRef"=w260) -> (reference out=w261:refnum<class "KeeperRoleVSS.lvclass">)  [unwired: 1 in, 1 out]
                n120 = Bundle By Name(cluster=w263, "KeeperRoleVSS"=w261) -> (w262:T9)
              }
              frame 2 {
                n121 = Unbundle By Name(w268) -> ("HaltRole A"=w269:refnum<class "HaltRole.lvclass">)
                n122 = property class="HaltRole"(reference=w269, "RobotRef"=w265) -> (reference out=w266:refnum<class "HaltRole.lvclass">)  [unwired: 1 in, 1 out]
                n123 = Bundle By Name(cluster=w268, "HaltRole A"=w266) -> (w267:T9)
              }
              frame 3 {
                n124 = Unbundle By Name(w273) -> ("HaltRole D"=w274:refnum<class "HaltRole.lvclass">)
                n125 = property class="HaltRole"(reference=w274, "RobotRef"=w270) -> (reference out=w271:refnum<class "HaltRole.lvclass">)  [unwired: 1 in, 1 out]
                n126 = Bundle By Name(cluster=w273, "HaltRole D"=w271) -> (w272:T9)
              }
            }
            n127 = property class="KickoffEnemyPlayVSS"(reference=w257, "Roles"=w258) -> (reference out=w256:refnum<class "KickoffEnemyPlayVSS.lvclass">)  [unwired: 1 in, 1 out]
            n128 = Bundle By Name(cluster=w249, "KickoffEnemyPlayVSS"=w256) -> (w245:T3)
            n129 = property class="Playbook"(reference=w255, "vss_plays"=w245) -> (reference out=w254:refnum<class "Playbook.lvclass">)  [unwired: 1 in, 1 out]
          }
        }
        frame "FreeBall" {
          n130 = property class="Playbook"(reference=w285) -> (reference out=w281:refnum<class "Playbook.lvclass">, "vss_plays"=w284:T3)  [unwired: 1 in, 1 out]
          n131 = call "pickVSSTeam.vi"("Ally in"=w279, "OldVSSTeam"=w280, "RobotRef"=w278, "Game"=w277) -> ("Ally out"=w275:refnum<class "Ally.lvclass">, "RobotRef Out"=w276:refnum<class "Robot.lvclass">[])  [unwired: 4 in, 1 out]
          n132 = for {
            tunnel: [w288] -> w282 mode=indexing
            tunnel: w276 -> [w293] mode=indexing
            shift-right: [w295] -> w283
            shift-left: w281 -> [w296]
            shift-right: [w286] -> _
            shift-left: w284 -> [w290]
            i -> [w292]
            n133 = Unbundle By Name(w290) -> ("FreeBallPlayVSS"=w289:refnum<class "FreeBallPlayVSS.lvclass">)
            n134 = property class="FreeBallPlayVSS"(reference=w289) -> (reference out=w298:refnum<class "FreeBallPlayVSS.lvclass">, "Roles"=w300:T4)  [unwired: 1 in, 1 out]
            n135 = Increment(x=w292) -> (x+1=w291:i32)
            n136 = property class="Robot"(reference=w293, "role"=roles."Timeout") -> (reference out=w287:refnum<class "Robot.lvclass">)  [unwired: 1 in, 1 out]
            n137 = case shown="3" w291 {
              tunnel: w300 -> [w304 w309 w314]
              tunnel: [w303 w308 w313] -> w299
              tunnel: w287 -> [w301 w306 w311]
              tunnel: [w301 w306 w311] -> w288
              frame 1, Default {
                n138 = Unbundle By Name(w304) -> ("KeeperRoleVSS"=w305:refnum<class "KeeperRoleVSS.lvclass">)
                n139 = property class="KeeperRoleVSS"(reference=w305, "RobotRef"=w301) -> (reference out=w302:refnum<class "KeeperRoleVSS.lvclass">)  [unwired: 1 in, 1 out]
                n140 = Bundle By Name(cluster=w304, "KeeperRoleVSS"=w302) -> (w303:T4)
              }
              frame 2 {
                n141 = Unbundle By Name(w309) -> ("NormalAttackerRoleVSS"=w310:refnum<class "NormalAttackerRoleVSS.lvclass">)
                n142 = property class="NormalAttackerRoleVSS"(reference=w310, "RobotRef"=w306) -> (reference out=w307:refnum<class "NormalAttackerRoleVSS.lvclass">)  [unwired: 1 in, 1 out]
                n143 = Bundle By Name(cluster=w309, "NormalAttackerRoleVSS"=w307) -> (w308:T4)
              }
              frame 3 {
                n144 = Unbundle By Name(w314) -> ("DefenderAreaRoleVSS"=w315:refnum<class "DefenderAreaRoleVSS.lvclass">)
                n145 = property class="DefenderAreaRoleVSS"(reference=w315, "RobotRef"=w311) -> (reference out=w312:refnum<class "DefenderAreaRoleVSS.lvclass">)  [unwired: 1 in, 1 out]
                n146 = Bundle By Name(cluster=w314, "DefenderAreaRoleVSS"=w312) -> (w313:T4)
              }
            }
            n147 = property class="FreeBallPlayVSS"(reference=w298, "Roles"=w299) -> (reference out=w297:refnum<class "FreeBallPlayVSS.lvclass">)  [unwired: 1 in, 1 out]
            n148 = Bundle By Name(cluster=w290, "FreeBallPlayVSS"=w297) -> (w286:T3)
            n149 = property class="Playbook"(reference=w296, "vss_plays"=w286) -> (reference out=w295:refnum<class "Playbook.lvclass">)  [unwired: 1 in, 1 out]
          }
        }
        frame "PrepareFreeBall", "PrepareGoalKickEnemy", "PrepareGoalKickAlly", "PrepareKickoffEnemy".."PreparePenaltyEnemy", "PreparePenaltyAlly" {
          n150 = property class="Playbook"(reference=w326) -> (reference out=w322:refnum<class "Playbook.lvclass">, "vss_plays"=w325:T3)  [unwired: 1 in, 1 out]
          n151 = call "pickVSSTeam.vi"("Ally in"=w320, "OldVSSTeam"=w321, "RobotRef"=w319, "Game"=w318) -> ("Ally out"=w316:refnum<class "Ally.lvclass">, "RobotRef Out"=w317:refnum<class "Robot.lvclass">[])  [unwired: 4 in, 1 out]
          n152 = for {
            tunnel: [w329] -> w323 mode=indexing
            tunnel: w317 -> [w334] mode=indexing
            shift-right: [w336] -> w324
            shift-left: w322 -> [w337]
            shift-right: [w327] -> _
            shift-left: w325 -> [w331]
            i -> [w333]
            n153 = Unbundle By Name(w331) -> ("HaltPlay"=w330:refnum<class "HaltPlay.lvclass">)
            n154 = property class="HaltPlay"(reference=w330) -> (reference out=w339:refnum<class "HaltPlay.lvclass">, "Roles"=w341:T10)  [unwired: 1 in, 1 out]
            n155 = Increment(x=w333) -> (x+1=w332:i32)
            n156 = property class="Robot"(reference=w334, "role"=roles."Timeout") -> (reference out=w328:refnum<class "Robot.lvclass">)  [unwired: 1 in, 1 out]
            n157 = case shown="3" w332 {
              tunnel: w341 -> [w345 w350 w355]
              tunnel: [w344 w349 w354] -> w340
              tunnel: w328 -> [w342 w347 w352]
              tunnel: [w342 w347 w352] -> w329
              frame 1, Default {
                n158 = Unbundle By Name(w345) -> ("HaltRole 1"=w346:refnum<class "HaltRole.lvclass">)
                n159 = property class="HaltRole"(reference=w346, "RobotRef"=w342) -> (reference out=w343:refnum<class "HaltRole.lvclass">)  [unwired: 1 in, 1 out]
                n160 = Bundle By Name(cluster=w345, "HaltRole 1"=w343) -> (w344:T10)
              }
              frame 2 {
                n161 = Unbundle By Name(w350) -> ("HaltRole 2"=w351:refnum<class "HaltRole.lvclass">)
                n162 = property class="HaltRole"(reference=w351, "RobotRef"=w347) -> (reference out=w348:refnum<class "HaltRole.lvclass">)  [unwired: 1 in, 1 out]
                n163 = Bundle By Name(cluster=w350, "HaltRole 2"=w348) -> (w349:T10)
              }
              frame 3 {
                n164 = Unbundle By Name(w355) -> ("HaltRole 3"=w356:refnum<class "HaltRole.lvclass">)
                n165 = property class="HaltRole"(reference=w356, "RobotRef"=w352) -> (reference out=w353:refnum<class "HaltRole.lvclass">)  [unwired: 1 in, 1 out]
                n166 = Bundle By Name(cluster=w355, "HaltRole 3"=w353) -> (w354:T10)
              }
            }
            n167 = property class="HaltPlay"(reference=w339, "Roles"=w340) -> (reference out=w338:refnum<class "HaltPlay.lvclass">)  [unwired: 1 in, 1 out]
            n168 = Bundle By Name(cluster=w331, "HaltPlay"=w338) -> (w327:T3)
            n169 = property class="Playbook"(reference=w337, "vss_plays"=w327) -> (reference out=w336:refnum<class "Playbook.lvclass">)  [unwired: 1 in, 1 out]
          }
        }
        frame "KickPenaltyAlly" {
          n170 = property class="Playbook"(reference=w367) -> (reference out=w363:refnum<class "Playbook.lvclass">, "vss_plays"=w366:T3)  [unwired: 1 in, 1 out]
          n171 = call "pickVSSTeam.vi"("Ally in"=w361, "OldVSSTeam"=w362, "RobotRef"=w360, "Game"=w359) -> ("Ally out"=w357:refnum<class "Ally.lvclass">, "RobotRef Out"=w358:refnum<class "Robot.lvclass">[])  [unwired: 4 in, 1 out]
          n172 = for {
            tunnel: [w370] -> w364 mode=indexing
            tunnel: w358 -> [w375] mode=indexing
            shift-right: [w377] -> w365
            shift-left: w363 -> [w378]
            shift-right: [w368] -> _
            shift-left: w366 -> [w372]
            i -> [w374]
            n173 = Unbundle By Name(w372) -> ("KickPenaltyAllyPlayVSS"=w371:refnum<class "KickPenaltyAllyPlayVSS.lvclass">)
            n174 = property class="KickPenaltyAllyPlayVSS"(reference=w371) -> (reference out=w380:refnum<class "KickPenaltyAllyPlayVSS.lvclass">, "Roles"=w382:T11)  [unwired: 1 in, 1 out]
            n175 = Increment(x=w374) -> (x+1=w373:i32)
            n176 = property class="Robot"(reference=w375, "role"=roles."Timeout") -> (reference out=w369:refnum<class "Robot.lvclass">)  [unwired: 1 in, 1 out]
            n177 = case shown="3" w373 {
              tunnel: w382 -> [w386 w391 w396]
              tunnel: [w385 w390 w395] -> w381
              tunnel: w369 -> [w383 w388 w393]
              tunnel: [w383 w388 w393] -> w370
              frame 1, Default {
                n178 = Unbundle By Name(w386) -> ("HaltRole K"=w387:refnum<class "HaltRole.lvclass">)
                n179 = property class="HaltRole"(reference=w387, "RobotRef"=w383) -> (reference out=w384:refnum<class "HaltRole.lvclass">)  [unwired: 1 in, 1 out]
                n180 = Bundle By Name(cluster=w386, "HaltRole K"=w384) -> (w385:T11)
              }
              frame 2 {
                n181 = Unbundle By Name(w391) -> ("NormalAttackerRoleVSS"=w392:refnum<class "NormalAttackerRoleVSS.lvclass">)
                n182 = property class="NormalAttackerRoleVSS"(reference=w392, "RobotRef"=w388) -> (reference out=w389:refnum<class "NormalAttackerRoleVSS.lvclass">)  [unwired: 1 in, 1 out]
                n183 = Bundle By Name(cluster=w391, "NormalAttackerRoleVSS"=w389) -> (w390:T11)
              }
              frame 3 {
                n184 = Unbundle By Name(w396) -> ("HaltRole D"=w397:refnum<class "HaltRole.lvclass">)
                n185 = property class="HaltRole"(reference=w397, "RobotRef"=w393) -> (reference out=w394:refnum<class "HaltRole.lvclass">)  [unwired: 1 in, 1 out]
                n186 = Bundle By Name(cluster=w396, "HaltRole D"=w394) -> (w395:T11)
              }
            }
            n187 = property class="KickPenaltyAllyPlayVSS"(reference=w380, "Roles"=w381) -> (reference out=w379:refnum<class "KickPenaltyAllyPlayVSS.lvclass">)  [unwired: 1 in, 1 out]
            n188 = Bundle By Name(cluster=w372, "KickPenaltyAllyPlayVSS"=w379) -> (w368:T3)
            n189 = property class="Playbook"(reference=w378, "vss_plays"=w368) -> (reference out=w377:refnum<class "Playbook.lvclass">)  [unwired: 1 in, 1 out]
          }
        }
        frame "DeadBall" {
          n190 = property class="Playbook"(reference=w408) -> (reference out=w404:refnum<class "Playbook.lvclass">, "vss_plays"=w407:T3)  [unwired: 1 in, 1 out]
          n191 = call "pickVSSTeam.vi"("Ally in"=w402, "OldVSSTeam"=w403, "RobotRef"=w401, "Game"=w400) -> ("Ally out"=w398:refnum<class "Ally.lvclass">, "RobotRef Out"=w399:refnum<class "Robot.lvclass">[])  [unwired: 4 in, 1 out]
          n192 = for {
            tunnel: [w411] -> w405 mode=indexing
            tunnel: w399 -> [w416] mode=indexing
            shift-right: [w418] -> w406
            shift-left: w404 -> [w419]
            shift-right: [w409] -> _
            shift-left: w407 -> [w413]
            i -> [w415]
            n193 = Unbundle By Name(w413) -> ("DeadBallPlayVSS"=w412:refnum<class "DeadBallPlayVSS.lvclass">)
            n194 = property class="DeadBallPlayVSS"(reference=w412) -> (reference out=w421:refnum<class "DeadBallPlayVSS.lvclass">, "Roles"=w423:T4)  [unwired: 1 in, 1 out]
            n195 = Increment(x=w415) -> (x+1=w414:i32)
            n196 = property class="Robot"(reference=w416, "role"=roles."Timeout") -> (reference out=w410:refnum<class "Robot.lvclass">)  [unwired: 1 in, 1 out]
            n197 = case shown="3" w414 {
              tunnel: w423 -> [w427 w432 w437]
              tunnel: [w426 w431 w436] -> w422
              tunnel: w410 -> [w424 w429 w434]
              tunnel: [w424 w429 w434] -> w411
              frame 1, Default {
                n198 = Unbundle By Name(w427) -> ("KeeperRoleVSS"=w428:refnum<class "KeeperRoleVSS.lvclass">)
                n199 = property class="KeeperRoleVSS"(reference=w428, "RobotRef"=w424) -> (reference out=w425:refnum<class "KeeperRoleVSS.lvclass">)  [unwired: 1 in, 1 out]
                n200 = Bundle By Name(cluster=w427, "KeeperRoleVSS"=w425) -> (w426:T4)
              }
              frame 2 {
                n201 = Unbundle By Name(w432) -> ("NormalAttackerRoleVSS"=w433:refnum<class "NormalAttackerRoleVSS.lvclass">)
                n202 = property class="NormalAttackerRoleVSS"(reference=w433, "RobotRef"=w429) -> (reference out=w430:refnum<class "NormalAttackerRoleVSS.lvclass">)  [unwired: 1 in, 1 out]
                n203 = Bundle By Name(cluster=w432, "NormalAttackerRoleVSS"=w430) -> (w431:T4)
              }
              frame 3 {
                n204 = Unbundle By Name(w437) -> ("DefenderAreaRoleVSS"=w438:refnum<class "DefenderAreaRoleVSS.lvclass">)
                n205 = property class="DefenderAreaRoleVSS"(reference=w438, "RobotRef"=w434) -> (reference out=w435:refnum<class "DefenderAreaRoleVSS.lvclass">)  [unwired: 1 in, 1 out]
                n206 = Bundle By Name(cluster=w437, "DefenderAreaRoleVSS"=w435) -> (w436:T4)
              }
            }
            n207 = property class="DeadBallPlayVSS"(reference=w421, "Roles"=w422) -> (reference out=w420:refnum<class "DeadBallPlayVSS.lvclass">)  [unwired: 1 in, 1 out]
            n208 = Bundle By Name(cluster=w413, "DeadBallPlayVSS"=w420) -> (w409:T3)
            n209 = property class="Playbook"(reference=w419, "vss_plays"=w409) -> (reference out=w418:refnum<class "Playbook.lvclass">)  [unwired: 1 in, 1 out]
          }
        }
        frame "PenaltyEnemy" {
          n210 = property class="Playbook"(reference=w449) -> (reference out=w445:refnum<class "Playbook.lvclass">, "vss_plays"=w448:T3)  [unwired: 1 in, 1 out]
          n211 = call "pickVSSTeam.vi"("Ally in"=w443, "OldVSSTeam"=w444, "RobotRef"=w442, "Game"=w441) -> ("Ally out"=w439:refnum<class "Ally.lvclass">, "RobotRef Out"=w440:refnum<class "Robot.lvclass">[])  [unwired: 4 in, 1 out]
          n212 = for {
            tunnel: [w452] -> w446 mode=indexing
            tunnel: w440 -> [w457] mode=indexing
            shift-right: [w459] -> w447
            shift-left: w445 -> [w460]
            shift-right: [w450] -> _
            shift-left: w448 -> [w454]
            i -> [w456]
            n213 = Unbundle By Name(w454) -> ("PenaltyEnemyPlayVSS"=w453:refnum<class "PenaltyEnemyPlayVSS.lvclass">)
            n214 = property class="PenaltyEnemyPlayVSS"(reference=w453) -> (reference out=w462:refnum<class "PenaltyEnemyPlayVSS.lvclass">, "Roles"=w464:T9)  [unwired: 1 in, 1 out]
            n215 = Increment(x=w456) -> (x+1=w455:i32)
            n216 = property class="Robot"(reference=w457, "role"=roles."Timeout") -> (reference out=w451:refnum<class "Robot.lvclass">)  [unwired: 1 in, 1 out]
            n217 = case shown="3" w455 {
              tunnel: w464 -> [w468 w473 w478]
              tunnel: [w467 w472 w477] -> w463
              tunnel: w451 -> [w465 w470 w475]
              tunnel: [w465 w470 w475] -> w452
              frame 1, Default {
                n218 = Unbundle By Name(w468) -> ("KeeperRoleVSS"=w469:refnum<class "KeeperRoleVSS.lvclass">)
                n219 = property class="KeeperRoleVSS"(reference=w469, "RobotRef"=w465) -> (reference out=w466:refnum<class "KeeperRoleVSS.lvclass">)  [unwired: 1 in, 1 out]
                n220 = Bundle By Name(cluster=w468, "KeeperRoleVSS"=w466) -> (w467:T9)
              }
              frame 2 {
                n221 = Unbundle By Name(w473) -> ("HaltRole A"=w474:refnum<class "HaltRole.lvclass">)
                n222 = property class="HaltRole"(reference=w474, "RobotRef"=w470) -> (reference out=w471:refnum<class "HaltRole.lvclass">)  [unwired: 1 in, 1 out]
                n223 = Bundle By Name(cluster=w473, "HaltRole A"=w471) -> (w472:T9)
              }
              frame 3 {
                n224 = Unbundle By Name(w478) -> ("HaltRole D"=w479:refnum<class "HaltRole.lvclass">)
                n225 = property class="HaltRole"(reference=w479, "RobotRef"=w475) -> (reference out=w476:refnum<class "HaltRole.lvclass">)  [unwired: 1 in, 1 out]
                n226 = Bundle By Name(cluster=w478, "HaltRole D"=w476) -> (w477:T9)
              }
            }
            n227 = property class="PenaltyEnemyPlayVSS"(reference=w462, "Roles"=w463) -> (reference out=w461:refnum<class "PenaltyEnemyPlayVSS.lvclass">)  [unwired: 1 in, 1 out]
            n228 = Bundle By Name(cluster=w454, "PenaltyEnemyPlayVSS"=w461) -> (w450:T3)
            n229 = property class="Playbook"(reference=w460, "vss_plays"=w450) -> (reference out=w459:refnum<class "Playbook.lvclass">)  [unwired: 1 in, 1 out]
          }
        }
        frame "BallChallenge" {
          n230 = property class="Playbook"(reference=w490) -> (reference out=w486:refnum<class "Playbook.lvclass">, "vss_plays"=w489:T3)  [unwired: 1 in, 1 out]
          n231 = call "pickVSSTeam.vi"("Ally in"=w484, "OldVSSTeam"=w485, "RobotRef"=w483, "Game"=w482) -> ("Ally out"=w480:refnum<class "Ally.lvclass">, "RobotRef Out"=w481:refnum<class "Robot.lvclass">[])  [unwired: 4 in, 1 out]
          n232 = for {
            tunnel: [w493] -> w487 mode=indexing
            tunnel: w481 -> [w498] mode=indexing
            shift-right: [w500] -> w488
            shift-left: w486 -> [w501]
            shift-right: [w491] -> _
            shift-left: w489 -> [w495]
            i -> [w497]
            n233 = Unbundle By Name(w495) -> ("BallChallengePlayVSS"=w494:refnum<class "BallChallengePlayVSS.lvclass">)
            n234 = property class="BallChallengePlayVSS"(reference=w494) -> (reference out=w503:refnum<class "BallChallengePlayVSS.lvclass">, "Roles"=w505:T12)  [unwired: 1 in, 1 out]
            n235 = Increment(x=w497) -> (x+1=w496:i32)
            n236 = property class="Robot"(reference=w498, "role"=roles."Timeout") -> (reference out=w492:refnum<class "Robot.lvclass">)  [unwired: 1 in, 1 out]
            n237 = case shown="1, Default" w496 {
              tunnel: w505 -> [w509 w514 w519]
              tunnel: [w508 w513 w518] -> w504
              tunnel: w492 -> [w506 w511 w516]
              tunnel: [w506 w511 w516] -> w493
              frame 1, Default {
                n238 = Unbundle By Name(w509) -> ("HaltRole 1"=w510:refnum<class "HaltRole.lvclass">)
                n239 = property class="HaltRole"(reference=w510, "RobotRef"=w506) -> (reference out=w507:refnum<class "HaltRole.lvclass">)  [unwired: 1 in, 1 out]
                n240 = Bundle By Name(cluster=w509, "HaltRole 1"=w507) -> (w508:T12)
              }
              frame 2 {
                n241 = Unbundle By Name(w514) -> ("BallChallengerAttackerRoleVSS"=w515:refnum<class "BallChallengerAttackerRoleVSS.lvclass">)
                n242 = property class="BallChallengerAttackerRoleVSS"(reference=w515, "RobotRef"=w511) -> (reference out=w512:refnum<class "BallChallengerAttackerRoleVSS.lvclass">)  [unwired: 1 in, 1 out]
                n243 = Bundle By Name(cluster=w514, "BallChallengerAttackerRoleVSS"=w512) -> (w513:T12)
              }
              frame 3 {
                n244 = Unbundle By Name(w519) -> ("HaltRole 2"=w520:refnum<class "HaltRole.lvclass">)
                n245 = property class="HaltRole"(reference=w520, "RobotRef"=w516) -> (reference out=w517:refnum<class "HaltRole.lvclass">)  [unwired: 1 in, 1 out]
                n246 = Bundle By Name(cluster=w519, "HaltRole 2"=w517) -> (w518:T12)
              }
            }
            n247 = property class="BallChallengePlayVSS"(reference=w503, "Roles"=w504) -> (reference out=w502:refnum<class "BallChallengePlayVSS.lvclass">)  [unwired: 1 in, 1 out]
            n248 = Bundle By Name(cluster=w495, "BallChallengePlayVSS"=w502) -> (w491:T3)
            n249 = property class="Playbook"(reference=w501, "vss_plays"=w491) -> (reference out=w500:refnum<class "Playbook.lvclass">)  [unwired: 1 in, 1 out]
          }
        }
        frame "Timeout" {
          n250 = property class="Playbook"(reference=w531) -> (reference out=w527:refnum<class "Playbook.lvclass">, "vss_plays"=w530:T3)  [unwired: 1 in, 1 out]
          n251 = call "pickVSSTeam.vi"("Ally in"=w525, "OldVSSTeam"=w526, "RobotRef"=w524, "Game"=w523) -> ("Ally out"=w521:refnum<class "Ally.lvclass">, "RobotRef Out"=w522:refnum<class "Robot.lvclass">[])  [unwired: 4 in, 1 out]
          n252 = for {
            tunnel: [w534] -> w528 mode=indexing
            tunnel: w522 -> [w539] mode=indexing
            shift-right: [w541] -> w529
            shift-left: w527 -> [w542]
            shift-right: [w532] -> _
            shift-left: w530 -> [w536]
            i -> [w538]
            n253 = Unbundle By Name(w536) -> ("TimeoutPlay"=w535:refnum<class "TimeoutPlay.lvclass">)
            n254 = property class="TimeoutPlay"(reference=w535) -> (reference out=w544:refnum<class "TimeoutPlay.lvclass">, "Roles"=w546:T13)  [unwired: 1 in, 1 out]
            n255 = Increment(x=w538) -> (x+1=w537:i32)
            n256 = property class="Robot"(reference=w539, "role"=roles."Timeout") -> (reference out=w533:refnum<class "Robot.lvclass">)  [unwired: 1 in, 1 out]
            n257 = case shown="2" w537 {
              tunnel: w546 -> [w550 w555 w560]
              tunnel: [w549 w554 w559] -> w545
              tunnel: w533 -> [w547 w552 w557]
              tunnel: [w547 w552 w557] -> w534
              frame 1, Default {
                n258 = Unbundle By Name(w550) -> ("TimeoutRole 1"=w551:refnum<class "TimeoutRole.lvclass">)
                n259 = property class="TimeoutRole"(reference=w551, "RobotRef"=w547) -> (reference out=w548:refnum<class "TimeoutRole.lvclass">)  [unwired: 1 in, 1 out]
                n260 = Bundle By Name(cluster=w550, "TimeoutRole 1"=w548) -> (w549:T13)
              }
              frame 2 {
                n261 = Unbundle By Name(w555) -> ("TimeoutRole 2"=w556:refnum<class "TimeoutRole.lvclass">)
                n262 = property class="TimeoutRole"(reference=w556, "RobotRef"=w552) -> (reference out=w553:refnum<class "TimeoutRole.lvclass">)  [unwired: 1 in, 1 out]
                n263 = Bundle By Name(cluster=w555, "TimeoutRole 1"=w553) -> (w554:T13)
              }
              frame 3 {
                n264 = Unbundle By Name(w560) -> ("TimeoutRole 3"=w561:refnum<class "TimeoutRole.lvclass">)
                n265 = property class="TimeoutRole"(reference=w561, "RobotRef"=w557) -> (reference out=w558:refnum<class "TimeoutRole.lvclass">)  [unwired: 1 in, 1 out]
                n266 = Bundle By Name(cluster=w560, "TimeoutRole 3"=w558) -> (w559:T13)
              }
            }
            n267 = property class="TimeoutPlay"(reference=w544, "Roles"=w545) -> (reference out=w543:refnum<class "TimeoutPlay.lvclass">)  [unwired: 1 in, 1 out]
            n268 = Bundle By Name(cluster=w536, "TimeoutPlay"=w543) -> (w532:T3)
            n269 = property class="Playbook"(reference=w542, "vss_plays"=w532) -> (reference out=w541:refnum<class "Playbook.lvclass">)  [unwired: 1 in, 1 out]
          }
        }
        frame "Halt" {
          n270 = property class="Playbook"(reference=w572) -> (reference out=w568:refnum<class "Playbook.lvclass">, "vss_plays"=w571:T3)  [unwired: 1 in, 1 out]
          n271 = call "pickVSSTeam.vi"("Ally in"=w566, "OldVSSTeam"=w567, "RobotRef"=w565, "Game"=w564) -> ("Ally out"=w562:refnum<class "Ally.lvclass">, "RobotRef Out"=w563:refnum<class "Robot.lvclass">[])  [unwired: 4 in, 1 out]
          n272 = for {
            tunnel: [w575] -> w569 mode=indexing
            tunnel: w563 -> [w580] mode=indexing
            shift-right: [w582] -> w570
            shift-left: w568 -> [w583]
            shift-right: [w573] -> _
            shift-left: w571 -> [w577]
            i -> [w579]
            n273 = Unbundle By Name(w577) -> ("HaltPlay"=w576:refnum<class "HaltPlay.lvclass">)
            n274 = property class="HaltPlay"(reference=w576) -> (reference out=w585:refnum<class "HaltPlay.lvclass">, "Roles"=w587:T10)  [unwired: 1 in, 1 out]
            n275 = Increment(x=w579) -> (x+1=w578:i32)
            n276 = property class="Robot"(reference=w580, "role"=roles."Halt") -> (reference out=w574:refnum<class "Robot.lvclass">)  [unwired: 1 in, 1 out]
            n277 = case shown="1, Default" w578 {
              tunnel: w587 -> [w591 w596 w601]
              tunnel: [w590 w595 w600] -> w586
              tunnel: w574 -> [w588 w593 w598]
              tunnel: [w588 w593 w598] -> w575
              frame 1, Default {
                n278 = Unbundle By Name(w591) -> ("HaltRole 1"=w592:refnum<class "HaltRole.lvclass">)
                n279 = property class="HaltRole"(reference=w592, "RobotRef"=w588) -> (reference out=w589:refnum<class "HaltRole.lvclass">)  [unwired: 1 in, 1 out]
                n280 = Bundle By Name(cluster=w591, "HaltRole 1"=w589) -> (w590:T10)
              }
              frame 2 {
                n281 = Unbundle By Name(w596) -> ("HaltRole 2"=w597:refnum<class "HaltRole.lvclass">)
                n282 = property class="HaltRole"(reference=w597, "RobotRef"=w593) -> (reference out=w594:refnum<class "HaltRole.lvclass">)  [unwired: 1 in, 1 out]
                n283 = Bundle By Name(cluster=w596, "HaltRole 2"=w594) -> (w595:T10)
              }
              frame 3 {
                n284 = Unbundle By Name(w601) -> ("HaltRole 3"=w602:refnum<class "HaltRole.lvclass">)
                n285 = property class="HaltRole"(reference=w602, "RobotRef"=w598) -> (reference out=w599:refnum<class "HaltRole.lvclass">)  [unwired: 1 in, 1 out]
                n286 = Bundle By Name(cluster=w601, "HaltRole 3"=w599) -> (w600:T10)
              }
            }
            n287 = property class="HaltPlay"(reference=w585, "Roles"=w586) -> (reference out=w584:refnum<class "HaltPlay.lvclass">)  [unwired: 1 in, 1 out]
            n288 = Bundle By Name(cluster=w577, "HaltPlay"=w584) -> (w573:T3)
            n289 = property class="Playbook"(reference=w583, "vss_plays"=w573) -> (reference out=w582:refnum<class "Playbook.lvclass">)  [unwired: 1 in, 1 out]
          }
        }
      }
      n290 = property class="Ally"(reference=w13, "RobotRef"=w11) -> (reference out=w14:refnum<class "Ally.lvclass">)  [unwired: 1 in, 1 out]
      n291 = property class="Game"(reference=w18, "KeeperTeam"=w14, "Playbook"=w17) -> (reference out=w16:refnum<class "Game.lvclass">)  [unwired: 1 in, 1 out]
    }
    frame Error {
    }
  }
  "error out" <- w3
  "Game out" <- w1
